vi "Amplitude Glide.vi"(5 "Amplitude":dbl=2000.0, 7 "Fs (Hz)":dbl=100000.0, 9 "Npts":i32) -> (6 "Y":dbl[](array[numeric]))   [LabVIEW 2015]
uses:
  <vilib>/Analysis/1siggen.llb/Ramp Pattern by Samples.vi
  <vilib>/Analysis/NI_AALBase.lvlib
panel:
  in  "reset signal":bool
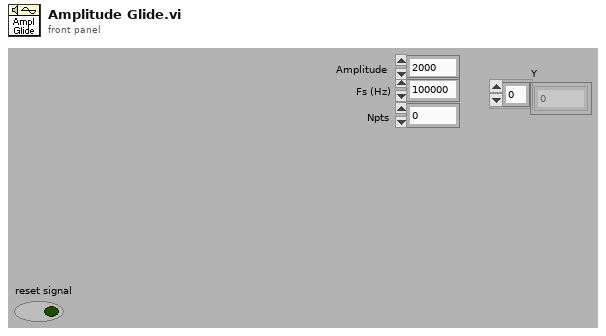
[diagram p1: front panel]
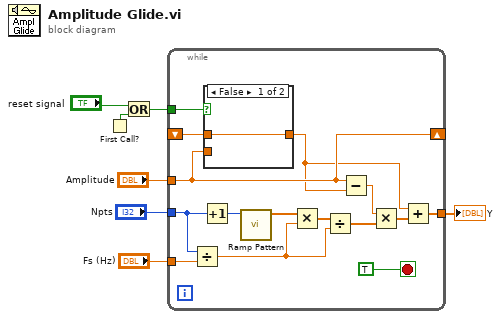
[diagram p0: block diagram]
diagram:
  n1 = First Call?() -> (First Call?: T/F=w3:bool)
  n2 = Or(x="reset signal", y=w3) -> (x .or. y?=w2:bool)
  n3 = while {
    tunnel: "Fs (Hz)" -> [w22]
    tunnel: "Npts" -> [w16]
    tunnel: "Amplitude" -> [w14]
    tunnel: [w10] -> w1
    tunnel: w2 -> [w8]
    shift-right: [w14] -> _
    shift-left: _ -> [w15]
    stop <- TRUE stop-if-true
    n4 = Divide(x=w16, y=w22) -> (x/y=w12:dbl)
    n5 = Increment(x=w16) -> (x+1=w18:i32)
    n6 = case shown="False" w8 {
      tunnel: w15 -> [w23 _]
      tunnel: [w23 w24] -> w9
      tunnel: w14 -> [_ w24]
      frame False {
      }
      frame True {
      }
    }
    n7 = call-poly <vilib>:"Ramp Pattern.vi"("samples"=w18) -> ("Ramp Pattern"=w21:dbl[])  [unwired: 9 in, 1 out]
    n8 = Multiply(x=w21, y=w12) -> (x*y=w13:dbl[])
    n9 = Divide(x=w13, y=w12) -> (x/y=w19:dbl[])
    n10 = Subtract(x=w14, y=w9) -> (x-y=w20:dbl)
    n11 = Multiply(x=w20, y=w19) -> (x*y=w11:dbl[])
    n12 = Add(x=w9, y=w11) -> (x+y=w10:dbl[])
  }
  "Y" <- w1
